vi "Wait for Convert.vi"(7 "1-Wire DIO Pin":refnum<k21>="ConnectorA/DIO15", 8 "error in":errorcluster) -> (0 "error out":errorcluster, 3 "Convert Time (usec)":u32)   [LabVIEW 2014, in "Maxim 1-Wire.lvlib"]
doc: "This VI is created by Vincent Claes for FPDA-1 more information on http://pwo.fpga.be\n\nvincent.claes@xios.be\nclaesvincent@gmail.com\n\nhttp://www.linkedin.com/in/vincentclaes"
uses:
  Maxim 1-Wire.lvlib
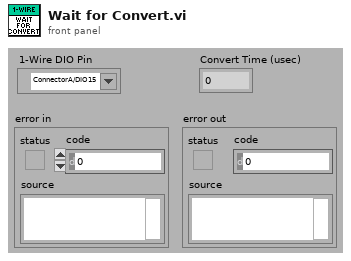
[diagram p1: front panel]
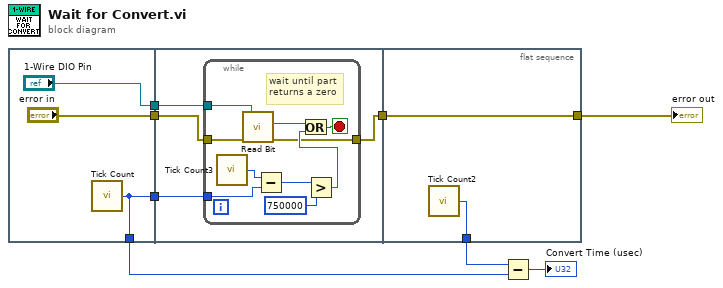
[diagram p0: block diagram]
diagram:
  n1 = flat-sequence {
    tunnel: ["error in"] -> w7
    tunnel: [w10] -> w4
    tunnel: [w10] -> w2
    tunnel: ["1-Wire DIO Pin"] -> w1
    tunnel: w7 -> [w15]
    tunnel: [w14] -> w6
    tunnel: w2 -> [w13]
    tunnel: w1 -> [w12]
    tunnel: [w27] -> w8
    tunnel: w6 -> [w27]
    tunnel: [w26] -> w5
    frame #0 {
      n2 = call "Tick Count"() -> ("Tick Count(uSec)"=w10:u32)
    }
    frame #1 {
      n3 = while {
        tunnel: w15 -> [w18]
        tunnel: [w17] -> w14
        tunnel: w13 -> [w24]
        tunnel: w12 -> [w19]
        stop <- w23 stop-if-true
        # "wait until part\nreturns a zero"
        n4 = call "Tick Count3"() -> ("Tick Count(uSec)"=w25:u32)
        n5 = call "Read Bit.vi"("1-Wire DIO Pin"=w19, "error in"=w18) -> ("error out"=w17:errorcluster, "Bit Read"=w16:bool)  [unwired: 8 in]
        n6 = Subtract(x=w25, y=w24) -> (x-y=w21:u32)
        n7 = Greater?(x=w21, y=u32 750000 ("x")) -> (0:w22:bool)
        n8 = Or(x=w16, y=w22) -> (x .or. y?=w23:bool)
      }
    }
    frame #2 {
      n9 = call "Tick Count2"() -> ("Tick Count(uSec)"=w26:u32)
    }
  }
  n10 = Subtract(x=w5, y=w4) -> (x-y=→"Convert Time (usec)":u32)
  "error out" <- w8
